vi "DockerTools - Parse container ID.vi"(7 "String (firefly-compose-app-1)":string="firefly-compose-app-1", 8 "Error In":errorcluster, 10 "Container list":string[][](array[string])) -> (0 "Error Out":errorcluster, 2 "Firefly iii App Container ID":string)   [LabVIEW 2017]
panel:
  in  "Multicolumn Listbox":i32(listbox)
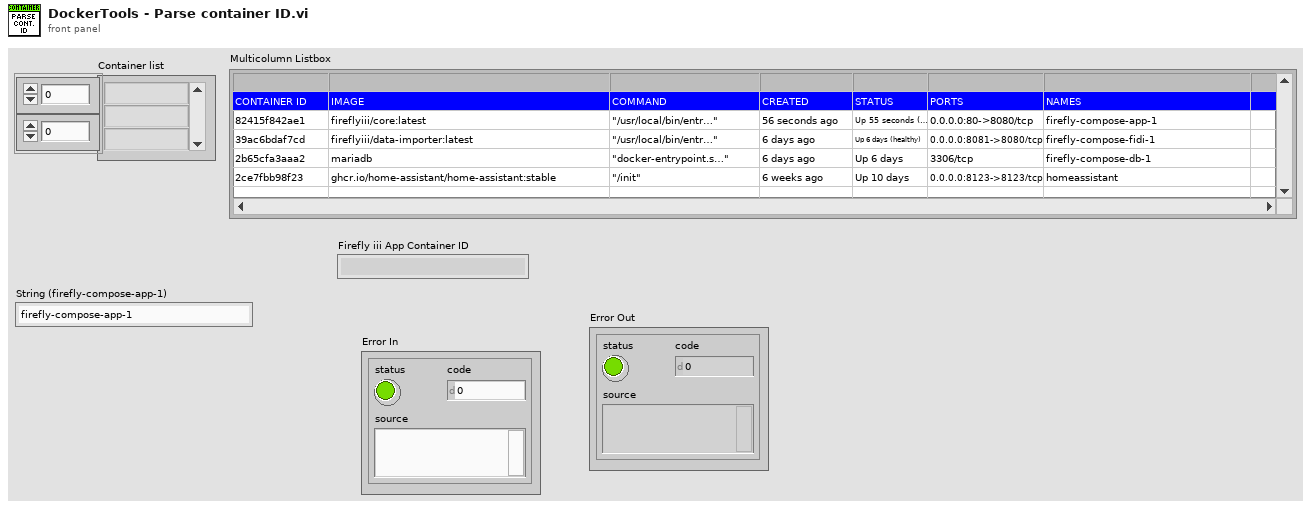
[diagram p1: front panel]
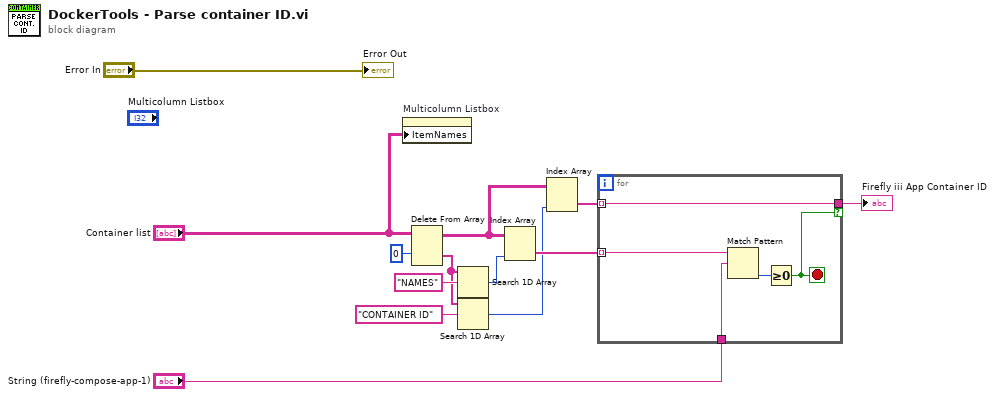
[diagram p0: block diagram]
diagram:
  n1 = property on="Multicolumn Listbox" class="MCListbox (strict)"("ItemNames"="Container list") -> ()  [unwired: 2 in, 2 out]
  n2 = Delete From Array(array="Container list", index (row)=0) -> (deleted portion=w8:string[], array with subset deleted=w7:string[][])  [unwired: 2 in]
  n3 = Search 1D Array(1D array=w8, element="NAMES") -> (index of element=w11:i32)  [unwired: 1 in]
  n4 = Search 1D Array(1D array=w8, element="CONTAINER ID") -> (index of element=w3:i32)  [unwired: 1 in]
  n5 = Index Array(array=w7, index (col)=w11) -> (element=w10:string[])  [unwired: 1 in]
  n6 = Index Array(array=w7, index (col)=w3) -> (element=w6:string[])  [unwired: 1 in]
  n7 = for {
    tunnel: w10 -> [w18] mode=indexing
    tunnel: w6 -> [w16] mode=indexing
    tunnel: [w16] -> w5 if=w15
    tunnel: "String (firefly-compose-app-1)" -> [w14]
    stop <- w15 stop-if-true
    n8 = Match Pattern(string=w18, regular expression=w14) -> (offset past match=w17:i32)  [unwired: 1 in, 3 out]
    n9 = Greater Or Equal To 0?(x=w17) -> (x >= 0?=w15:bool)
  }
  "Firefly iii App Container ID" <- w5
  "Error Out" <- "Error In"
